vi "state change logic.vi"(1 "mode set":T1, 2 "system state in":T2, 11 "exit":bool) -> (3 "system state out":T2, 8 "change state":bool, 15 "exit program":bool)   [LabVIEW 2016]
doc: "This Vi is were all the magic happens, it looks at the input to determine if is on auto, blinking or all test on mode, and based of that choose the appropiate mode and excetutes the code in each until another mode is call.\n\nAlexis Lopez\nP350\nCSUSB Physics"
uses:
  typedefs/system state cluster.ctl
  typedefs/state enum.ctl
  typedefs/control mode enum.ctl
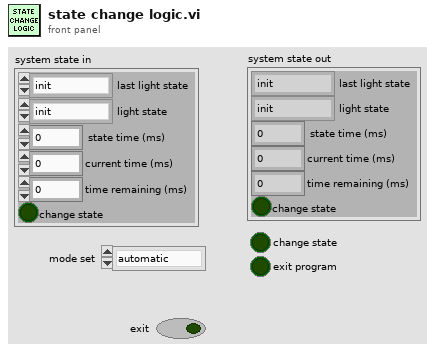
[diagram p1: front panel]
types:
  T1 = typedef "control mode enum.ctl" = enum16{"automatic", "blinking", "all on test"}
  T2 = typedef "system state cluster.ctl" = cluster{"last light state":T3, "light state":T3, "state time (ms)":i32, "current time (ms)":i32, "time remaining (ms)":i32, "change state":bool}
  T3 = typedef "state enum.ctl" = enum16{"init", "idle", "left turn E", "go EW", "caution EW", "left turn W", "left turn N", "go NS", "caution NS", "left turn S", "blink on", "blink off", "all on test", "exit"}
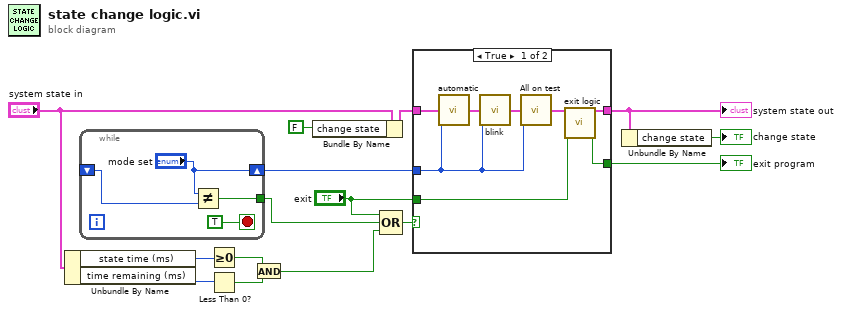
[diagram p0: block diagram]
diagram:
  n1 = Unbundle By Name("system state in") -> ("state time (ms)"=w7:i32, "time remaining (ms)"=w6:i32)
  n2 = while {
    shift-right: ["mode set"] -> w2
    shift-left: _ -> [w19]
    tunnel: [w17] -> w1
    stop <- TRUE stop-if-true
    n3 = Not Equal?(x="mode set", y=w19) -> (x != y?=w17:bool)
  }
  n4 = Greater Or Equal To 0?(x=w7) -> (x >= 0?=w5:bool)
  n5 = Less Than 0?(x=w6) -> (x < 0?=w4:bool)
  n6 = And(x=w5, y=w4) -> (x .and. y?=w3:bool)
  n7 = Bundle By Name(cluster="system state in", "change state"=FALSE) -> (w10:T2)
  n8 = Compound Arithmetic op=OR("exit", w1, w3) -> (w11:bool)
  n9 = case shown="True" w11 {
    tunnel: [w27 _] -> w15
    tunnel: [w26 w28] -> w14
    tunnel: w10 -> [w24 w28]
    tunnel: "exit" -> [w25 _]
    tunnel: w2 -> [w20 _]
    frame True {
      n10 = call "automatic.vi"("system state in"=w24, "mode set"=w20) -> ("system state out"=w23:T2)  [unwired: 13 in]
      n11 = call "blink.vi"("system state in"=w23, "mode set"=w20) -> ("system state out"=w22:T2)  [unwired: 13 in]
      n12 = call "All on test.vi"("system state in in"=w22, "mode set"=w20) -> ("system state out"=w21:T2)  [unwired: 13 in]
      n13 = call "exit logic.vi"("system state in"=w21, "exit"=w25) -> ("system state out"=w26:T2, "exit program"=w27:bool)  [unwired: 12 in]
    }
    frame False {
    }
  }
  "system state out" <- w14
  "exit program" <- w15
  n14 = Unbundle By Name(w14) -> ("change state"=→"change state":bool)
